vi "b-spline.vi"(6 "percision":dbl=0.01, 7 "weights":dbl[](array[numeric]), 8 "error in":errorcluster, 9 "knots":dbl[](array[numeric]), 10 "degree":u16, 11 "points":dbl[][](array[numeric])) -> (0 "error out":errorcluster, 3 "spline":dbl[][](array[numeric]))   [LabVIEW 2019]
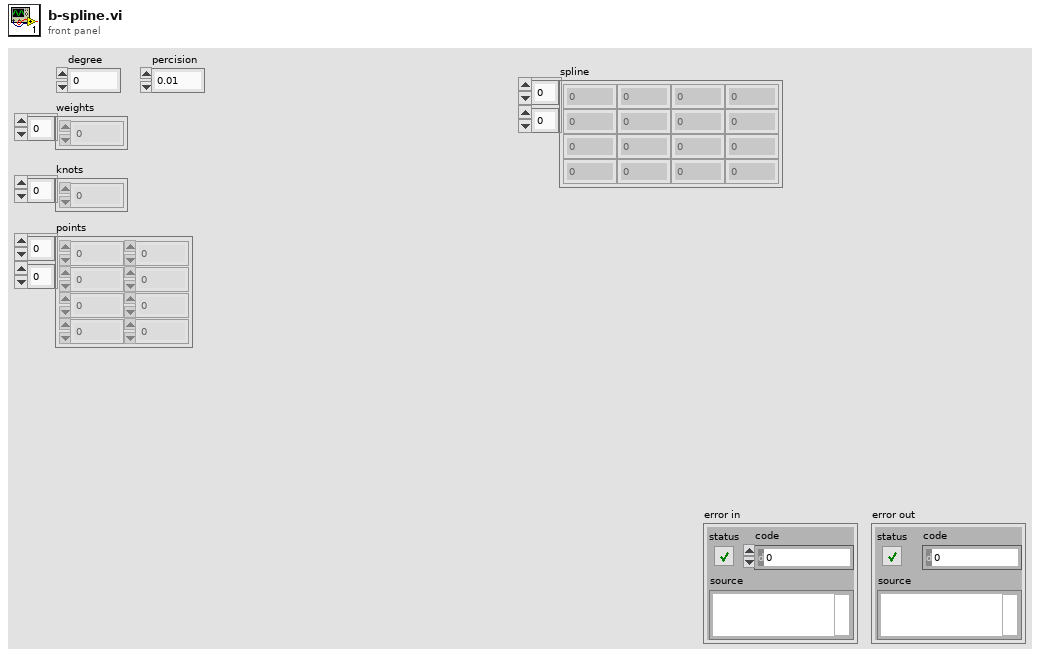
[diagram p1: front panel]
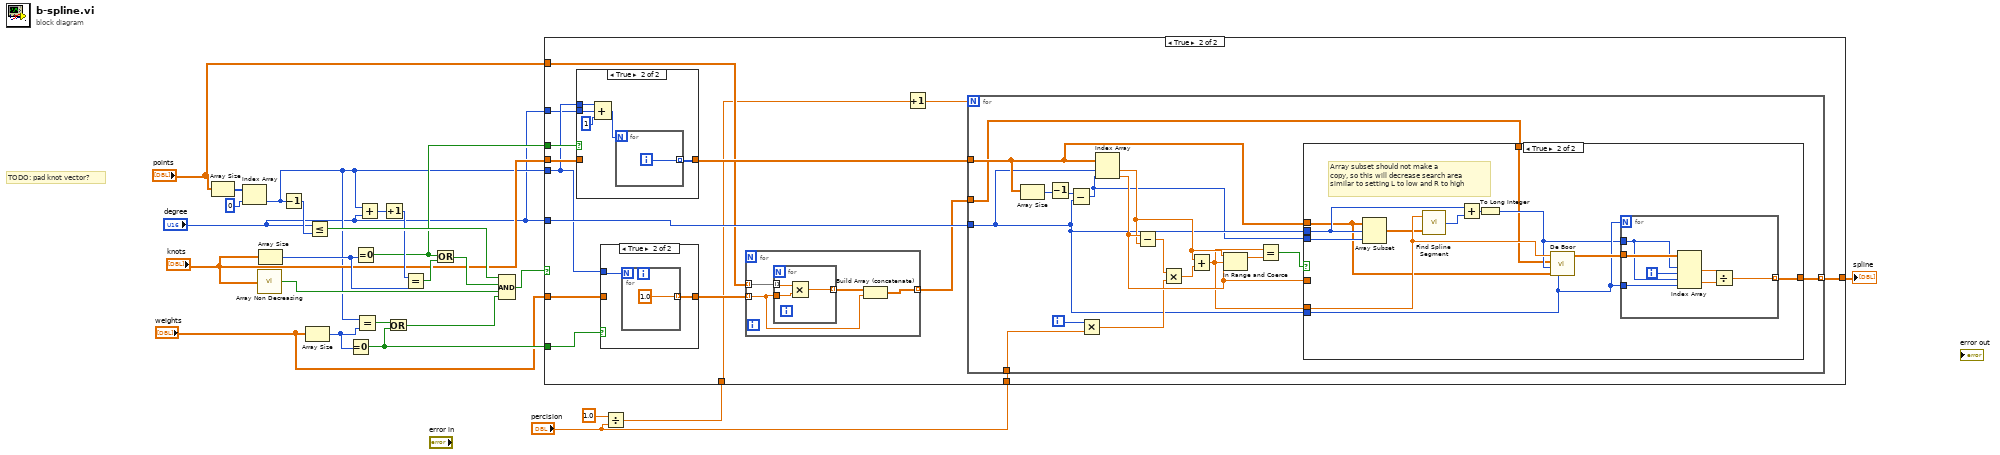
[diagram p0: block diagram]
diagram:
  # "TODO: pad knot vector?"
  n1 = Array Size(array="points") -> (size(s)=w6:i32[])
  n2 = Index Array(array=w6, index=0) -> (element=w5:i32)
  n3 = call "Array Non Decreasing.vi"("array"="knots") -> ("Non Decreasing?"=w22:bool)
  n4 = Array Size(array="knots") -> (size(s)=w14:i32)
  n5 = Decrement(x=w5) -> (x-1=w25:i32)
  n6 = Array Size(array="weights") -> (size(s)=w18:i32)
  n7 = Less Or Equal?(x="degree", y=w25) -> (x <= y?=w23:bool)
  n8 = Equal To 0?(x=w18) -> (x = 0?=w16:bool)
  n9 = Equal To 0?(x=w14) -> (x = 0?=w12:bool)
  n10 = Equal?(x=w5, y=w18) -> (x = y?=w19:bool)
  n11 = Add(x=w5, y="degree") -> (x+y=w21:i32)
  n12 = Increment(x=w21) -> (x+1=w20:i32)
  n13 = Or(x=w19, y=w16) -> (x .or. y?=w17:bool)
  n14 = Equal?(x=w20, y=w14) -> (x = y?=w15:bool)
  n15 = Or(x=w12, y=w15) -> (x .or. y?=w13:bool)
  n16 = Compound Arithmetic op=AND(w23, w13, w22, w17) -> (w24:bool)
  n17 = Divide(x=1.0, y="percision") -> (x/y=w9:dbl)
  n18 = case shown="True" w24 {
    tunnel: w16 -> [_ w40]
    tunnel: "weights" -> [_ w39]
    tunnel: w5 -> [_ w32]
    tunnel: w12 -> [_ w38]
    tunnel: "knots" -> [_ w37]
    tunnel: "points" -> [_ w29]
    tunnel: "degree" -> [_ w35]
    tunnel: w9 -> [_ w26]
    tunnel: "percision" -> [_ w34]
    tunnel: "degree" -> [_ w31]
    tunnel: [_ w30] -> w1
    frame False {
    }
    frame True {
      n19 = case shown="True" w38 {
        tunnel: w37 -> [w48 _]
        tunnel: [w48 w53] -> w36
        tunnel: w32 -> [_ w52]
        tunnel: w31 -> [_ w51]
        frame False {
        }
        frame True {
          n20 = Compound Arithmetic op=ADD(w52, w51, u16 1 ("value")) -> (w49:i32)
          n21 = for {
            N: w49 -> [_]
            tunnel: [w54] -> w53 mode=indexing
            i -> [w54]
          }
        }
      }
      n22 = case shown="True" w40 {
        tunnel: w39 -> [w55 _]
        tunnel: [w55 w56] -> w27
        tunnel: w32 -> [_ w57]
        frame False {
        }
        frame True {
          n23 = for {
            N: w57 -> [_]
            tunnel: [1.0] -> w56 mode=indexing
          }
        }
      }
      n24 = for {
        tunnel: w29 -> [w44] mode=indexing
        tunnel: w27 -> [w42] mode=indexing
        tunnel: [w41] -> w28 mode=indexing
        n25 = for {
          tunnel: w44 -> [w47] mode=indexing
          tunnel: w42 -> [w46]
          tunnel: [w45] -> w43 mode=indexing
          n26 = Multiply(x=w47, y=w46) -> (x*y=w45:dbl)
        }
        n27 = Build Array (concatenate)(w43, w42) -> (w41:dbl[])
      }
      n28 = Increment(x=w26) -> (x+1=w33:dbl)
      n29 = for {
        N: w33 -> [_]
        tunnel: w36 -> [w70]
        tunnel: w28 -> [w69]
        tunnel: w35 -> [w60]
        tunnel: w34 -> [w72]
        tunnel: [w68] -> w30 mode=indexing
        i -> [w73]
        n30 = Array Size(array=w70) -> (size(s)=w75:i32)
        n31 = Decrement(x=w75) -> (x-1=w74:i32)
        n32 = Subtract(x=w74, y=w60) -> (x-y=w59:i32)
        n33 = Multiply(x=w73, y=w72) -> (x*y=w63:dbl)
        n34 = Index Array(array=w70, index #1=w60, index #2=w59) -> (element #1=w66:dbl, element #2=w67:dbl)
        n35 = Subtract(x=w67, y=w66) -> (x-y=w61:dbl)
        n36 = Multiply(x=w61, y=w63) -> (x*y=w71:dbl)
        n37 = Add(x=w66, y=w71) -> (x+y=w62:dbl)
        n38 = In Range and Coerce(upper limit=w66, x=w62, lower limit=w67) -> (coerced(x)=w65:dbl)  [unwired: 1 out]
        n39 = Equal?(x=w62, y=w65) -> (x = y?=w64:bool)
        n40 = case shown="True" w64 {
          tunnel: w70 -> [_ w76]
          tunnel: w67 -> [_ _]
          tunnel: w62 -> [_ w87]
          tunnel: w69 -> [_ w77]
          tunnel: w60 -> [_ w85]
          tunnel: [_ w84] -> w68
          tunnel: w59 -> [_ w82]
          tunnel: w60 -> [_ w78]
          frame False {
          }
          frame True {
            # "Array subset should not make a\ncopy, so this will decrease search area\nsimilar to setting L to low and R to high"
            n41 = Array Subset(array=w76, index=w78, length=w82) -> (w83:dbl[])
            n42 = call "Find Spline Segment.vi"("knots"=w83, "t"=w87) -> ("spline segment idx"=w81:i32)
            n43 = Add(x=w78, y=w81) -> (x+y=w80:i32)
            n44 = To Long Integer(number=w80) -> (32bit integer=w79:i32)
            n45 = call "De Boor.vi"("degree"=w85, "knots"=w76, "spline segment idx"=w79, "points"=w77, "position"=w87) -> ("points out"=w86:dbl[][])  [unwired: 6 in]
            n46 = for {
              N: w85 -> [_]
              tunnel: w86 -> [w94]
              tunnel: w79 -> [w92]
              tunnel: w85 -> [w91]
              tunnel: [w88] -> w84 mode=indexing
              i -> [w93]
              n47 = Index Array(array=w94, index (row) #1=w92, index (col) #1=w93, index (row) #2=w92, index (col) #2=w91) -> (element #1=w89:dbl, element #2=w90:dbl)
              n48 = Divide(x=w89, y=w90) -> (x/y=w88:dbl)
            }
          }
        }
      }
    }
  }
  "spline" <- w1
